vi "ykgw_close.vi"(8 "error in (no error)":errorcluster, 10 "DestroyAll":bool, 11 "Instrument in":refnum<class "Instrument.lvclass">) -> (0 "error out":errorcluster, 3 "Instrument out":refnum<class "Instrument.lvclass">)   [LabVIEW 2019, in "Instrument.lvclass"]
uses:
  Instrument.lvclass
  Instrument.lvclass/Instrument.ctl
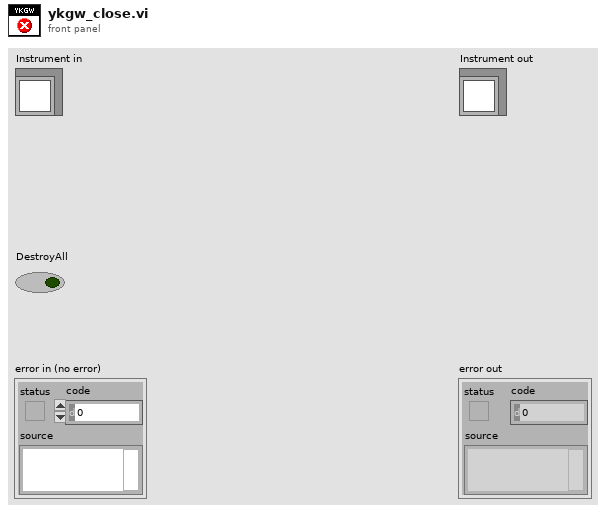
[diagram p1: front panel]
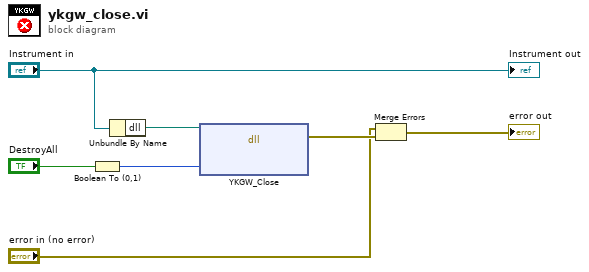
[diagram p0: block diagram]
diagram:
  n1 = Boolean To (0,1)(Boolean="DestroyAll") -> (0, 1=w1:i16)
  n2 = Unbundle By Name("Instrument in") -> ("dll"=w5:path)
  n3 = dll-call lib="C:/Dev/22KW-Dyno/software/data/DynoAPI.dll" fn="YKGW_Close"(path in=w5, "DestroyAll"=w1) -> (error out=w7:errorcluster)  [unwired: 4 in, 1 out]
  n4 = Merge Errors("error in (no error)", w7) -> (→"error out":errorcluster)
  "Instrument out" <- "Instrument in"
